vi "test01.vi"() -> ()   [LabVIEW 2019]
uses:
  <vilib>/myRIO/Instrument Drivers/Onboard IO/DIO/typedefs/DIO Reference.ctl
  <vilib>/myRIO/Common/Instrument Driver Framework/Utilities/typedefs/myRIO Generic Hardware Reference.ctl
  <vilib>/myRIO/Common/Instrument Driver Framework/Utilities/typedefs/Hardware Version Enum.ctl
  <vilib>/myRIO/Common/Instrument Driver Framework/Utilities/typedefs/myRIO v1.0 Reference.ctl
  <vilib>/myRIO/Common/Instrument Driver Framework/Utilities/typedefs/Generic FPGA Reference.ctl
  <vilib>/myRIO/Common/Instrument Driver Framework/myRIO v1.0/DIO/typedefs/DIO Channels List.ctl
  <vilib>/myRIO/Common/Instrument Driver Framework/myRIO v1.0/DIO/typedefs/DIO Channels Enum.ctl
  <vilib>/userDefined/High Color/nirio_resource_hc.ctl
  <vilib>/myRIO/Common/Instrument Driver Framework/Utilities/vis/Is FPGA Ref Available.vi
  <vilib>/myRIO/Common/Instrument Driver Framework/myRIO v1.0/DIO/vis/myRIO v1.1 Open DIO.vi
  <vilib>/myRIO/Instrument Drivers/Onboard IO/DIO/vis/Read.vi
  <vilib>/myRIO/Common/Instrument Driver Framework/myRIO v1.0/UART/vis/myRIO v1.0 Close UART.vi
  <vilib>/myRIO/Common/Instrument Driver Framework/Utilities/vis/Validate Channels.vi
  <vilib>/myRIO/Common/Instrument Driver Framework/myRIO v1.0/DIO/vis/myRIO v1.0 Reserve DIO.vi
  <vilib>/myRIO/Common/Instrument Driver Framework/myRIO v1.0/Resource Manager/vis/myRIO v1.0 Reserve Channel List.vi
  <vilib>/myRIO/Common/Instrument Driver Framework/myRIO v1.0/DIO/vis/myRIO v1.0 Build MUX Configuration DIO.vi
  <vilib>/myRIO/Common/Instrument Driver Framework/myRIO v1.0/Resource Manager/vis/myRIO v1.0 Reserve Channel.vi
  <vilib>/myRIO/Common/Instrument Driver Framework/myRIO v1.0/Resource Manager/vis/myRIO v1.0 Unreserve Channel.vi
  <vilib>/myRIO/Common/Instrument Driver Framework/myRIO v1.0/Resource Manager/vis/myRIO v1.0 Create Configuration List.vi
  <vilib>/myRIO/Common/Instrument Driver Framework/myRIO v1.0/Resource Manager/vis/myRIO v1.0 Build Mutex Name.vi
  <vilib>/myRIO/Common/Instrument Driver Framework/Utilities/vis/FPGA Ref Manager.vi
  <vilib>/myRIO/Common/Instrument Driver Framework/myRIO v1.0/myRIO v1.0 Reset FPGA.vi
  <vilib>/myRIO/Common/Instrument Driver Framework/myRIO v1.0/IRQ/vis/myRIO v1.0 IRQ Info FGV.vi
  <vilib>/myRIO/Common/Instrument Driver Framework/myRIO v1.0/IRQ/vis/myRIO v1.0 Timer IRQ Info FGV.vi
  <vilib>/myRIO/Common/Instrument Driver Framework/myRIO v1.0/IRQ/vis/myRIO v1.0 ISR Agent.vi
  <vilib>/myRIO/Instrument Drivers/Utilities/vis/Reset Index.vi
  <vilib>/myRIO/Common/Instrument Driver Framework/myRIO v1.0/Resource Manager/vis/myRIO v1.0 Block Write Resource Manager.vi
  <vilib>/Utility/VariantDataType/GetNumericInfo.vi
  <vilib>/Utility/error.llb/Error Cluster From Error Code.vi
  <vilib>/myRIO/Common/Instrument Driver Framework/myRIO v1.0/myRIO v1.1 Open.vi
  <vilib>/myRIO/Common/Instrument Driver Framework/Utilities/vis/IO Manager.vi
  <vilib>/myRIO/Common/Instrument Driver Framework/Utilities/vis/Configuration Manager.vi
  <vilib>/myRIO/Common/Instrument Driver Framework/myRIO v1.0/Resource Manager/vis/myRIO v1.0 Configure IO.vi
  <vilib>/myRIO/Common/Instrument Driver Framework/myRIO v1.0/myRIO v1.0 Close.vi
  <vilib>/myRIO/Common/Instrument Driver Framework/myRIO v1.0/DIO/vis/myRIO v1.0 Read DIO.vi
  <vilib>/myRIO/Express VI/Onboard Devices/Button/Button Express VI.xnode
  <vilib>/myRIO/Instrument Drivers/Onboard IO/DIO/vis/myRIO DIO Open.xnode
  <vilib>/myRIO/Instrument Drivers/Onboard IO/DIO/DIO.lvlib
  <vilib>/myRIO/Instrument Drivers/Utilities/Utilities.lvlib
panel:
  out "error out":errorcluster
  in  "error in (no error)":errorcluster
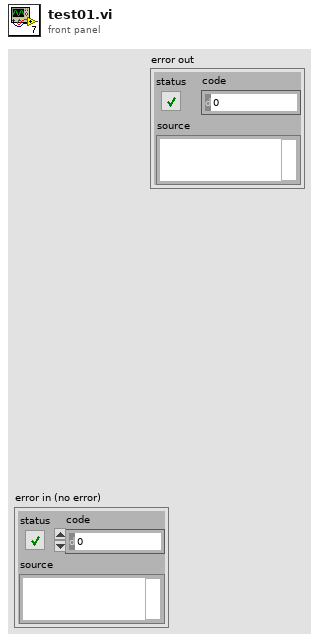
[diagram p1: front panel]
types:
  T1 = typedef "DIO.lvlib/DIO Reference.ctl" = cluster{"myRIO Reference":T2, "DIO Channels List":T6}
  T2 = typedef "myRIO Generic Hardware Reference.ctl" = cluster{"myRIO Model":T3, "myRIO Hardware Reference":T4}
  T3 = typedef "Hardware Version Enum.ctl" = enum16{"Unknown", "myRIO-1900", "myRIO-1950", "roboRIO", "NI ELVIS RIO CM", "ELVIS III"}
  T4 = typedef "myRIO v1.0 Reference.ctl" = cluster{"Generic FPGA Reference":T5, "Allow multiple opens":bool}
  T5 = typedef "Generic FPGA Reference.ctl" = refnum<k20>
  T6 = typedef "DIO Channels List.ctl" = T7[]
  T7 = typedef "DIO Channels Enum.ctl" = enum16{"Not Connected", "C/DIO0", "C/DIO1", "C/DIO2", "C/DIO3", "C/DIO4", "C/DIO5", "C/DIO6", "C/DIO7", "A/DIO0", "A/DIO1", "A/DIO2", "A/DIO3", "A/DIO4", "A/DIO5", "A/DIO6", "A/DIO7", "A/DIO8", "A/DIO9", "A/DIO10", "A/DIO11", "A/DIO12", "A/DIO13", "A/DIO14", "A/DIO15", "A/DIO16", "A/DIO17", "A/DIO18", "A/DIO19", "B/DIO0", "B/DIO1", "B/DIO2", "B/DIO3", "B/DIO4", "B/DIO5", "B/DIO6", "B/DIO7", "B/DIO8", "B/DIO9", "B/DIO10", "B/DIO11", "B/DIO12", "B/DIO13", "B/DIO14", "B/DIO15", "B/DIO16", "B/DIO17", "B/DIO18", "B/DIO19", "LED0", "LED1", "LED2", "LED3", "Button0", "DIO/DIO0", "DIO/DIO1", "DIO/DIO2", "DIO/DIO3", "DIO/DIO4", "DIO/DIO5", "DIO/DIO6", "DIO/DIO7", "DIO/DIO8", "DIO/DIO9", "SPI/CS0", "SPI/CS1", "SPI/CS2", "SPI/CS3", "LED RADIO (Green)", "LED RADIO (Red)", "LED COMM (Green)", "LED COMM (Red)", "LED MODE (Green)", "LED MODE (Red)"}
  T8 = typedef "nirio_resource_hc.ctl" = tag
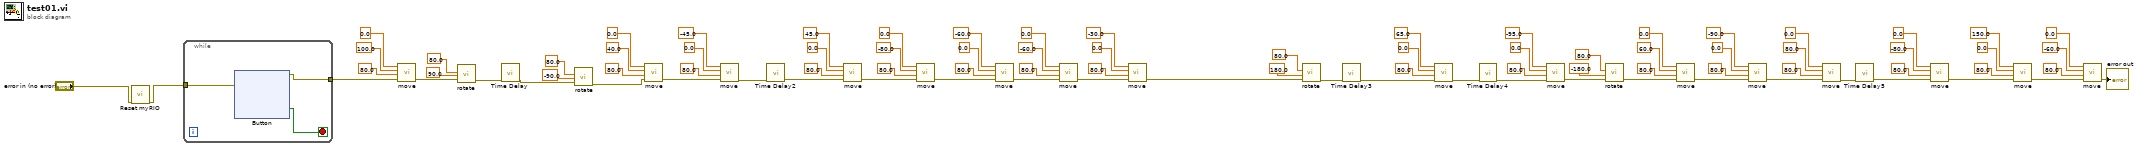
[diagram p0: block diagram]
diagram:
  n1 = call <vilib>:"Reset myRIO.vi"("error in (no error)"="error in (no error)") -> ("error out"=w7:errorcluster)  [unwired: 10 in]
  n2 = while {
    tunnel: [w86] -> w8
    tunnel: w7 -> [w85]
    stop <- w87 stop-if-true
    n3 = xnode "Button"("error in (no error)"=w85) -> ("Value"=w87:bool, "error out"=w86:errorcluster)
  }
  n4 = call "move.vi"("error in (no error)"=w8, "RPM"=80.0, "y"=100.0, "X"=0.0) -> ("error out"=w84:errorcluster)  [unwired: 7 in]
  n5 = call "rotate.vi"("error in (no error)"=w84, "speed"=80.0, "degree"=90.0) -> ("error out"=w78:errorcluster)  [unwired: 8 in]
  n6 = call "Time Delay"("error in (no error)"=w78) -> ("error out"=w75:errorcluster)  [unwired: 10 in]
  n7 = call "rotate.vi"("error in (no error)"=w75, "speed"=80.0, "degree"=-90.0) -> ("error out"=w72:errorcluster)  [unwired: 8 in]
  n8 = call "move.vi"("error in (no error)"=w72, "RPM"=80.0, "y"=40.0, "X"=0.0) -> ("error out"=w67:errorcluster)  [unwired: 7 in]
  n9 = call "move.vi"("error in (no error)"=w67, "RPM"=80.0, "y"=0.0, "X"=-45.0) -> ("error out"=w66:errorcluster)  [unwired: 7 in]
  n10 = call "Time Delay2"("error in (no error)"=w66) -> ("error out"=w62:errorcluster)  [unwired: 10 in]
  n11 = call "move.vi"("error in (no error)"=w62, "RPM"=80.0, "y"=0.0, "X"=45.0) -> ("error out"=w58:errorcluster)  [unwired: 7 in]
  n12 = call "move.vi"("error in (no error)"=w58, "RPM"=80.0, "y"=-80.0, "X"=0.0) -> ("error out"=w54:errorcluster)  [unwired: 7 in]
  n13 = call "move.vi"("error in (no error)"=w54, "RPM"=80.0, "y"=0.0, "X"=-60.0) -> ("error out"=w50:errorcluster)  [unwired: 7 in]
  n14 = call "move.vi"("error in (no error)"=w50, "RPM"=80.0, "y"=-60.0, "X"=0.0) -> ("error out"=w2:errorcluster)  [unwired: 7 in]
  n15 = call "move.vi"("error in (no error)"=w2, "RPM"=80.0, "y"=0.0, "X"=-30.0) -> ("error out"=w1:errorcluster)  [unwired: 7 in]
  n16 = call "rotate.vi"("error in (no error)"=w1, "speed"=80.0, "degree"=180.0) -> ("error out"=w44:errorcluster)  [unwired: 8 in]
  n17 = call "Time Delay3"("error in (no error)"=w44) -> ("error out"=w43:errorcluster)  [unwired: 10 in]
  n18 = call "move.vi"("error in (no error)"=w43, "RPM"=80.0, "y"=0.0, "X"=65.0) -> ("error out"=w42:errorcluster)  [unwired: 7 in]
  n19 = call "Time Delay4"("error in (no error)"=w42) -> ("error out"=w38:errorcluster)  [unwired: 10 in]
  n20 = call "move.vi"("error in (no error)"=w38, "RPM"=80.0, "y"=0.0, "X"=-95.0) -> ("error out"=w35:errorcluster)  [unwired: 7 in]
  n21 = call "rotate.vi"("error in (no error)"=w35, "speed"=80.0, "degree"=-180.0) -> ("error out"=w31:errorcluster)  [unwired: 8 in]
  n22 = call "move.vi"("error in (no error)"=w31, "RPM"=80.0, "y"=60.0, "X"=0.0) -> ("error out"=w27:errorcluster)  [unwired: 7 in]
  n23 = call "move.vi"("error in (no error)"=w27, "RPM"=80.0, "y"=0.0, "X"=-90.0) -> ("error out"=w23:errorcluster)  [unwired: 7 in]
  n24 = call "move.vi"("error in (no error)"=w23, "RPM"=80.0, "y"=80.0, "X"=0.0) -> ("error out"=w22:errorcluster)  [unwired: 7 in]
  n25 = call "Time Delay5"("error in (no error)"=w22) -> ("error out"=w18:errorcluster)  [unwired: 10 in]
  n26 = call "move.vi"("error in (no error)"=w18, "RPM"=80.0, "y"=-80.0, "X"=0.0) -> ("error out"=w14:errorcluster)  [unwired: 7 in]
  n27 = call "move.vi"("error in (no error)"=w14, "RPM"=80.0, "y"=0.0, "X"=150.0) -> ("error out"=w10:errorcluster)  [unwired: 7 in]
  n28 = call "move.vi"("error in (no error)"=w10, "RPM"=80.0, "y"=-60.0, "X"=0.0) -> ("error out"=→"error out":errorcluster)  [unwired: 7 in]
